vi "value to ring (SequenceNumberOffset).vi"(11 "value":string) -> (3 "SequenceNumberOffset":T1=65535 items=["FDX_TX_FRAME_SEQ_OFFS_AUTO"=65535])   [LabVIEW 2020, in "AIM ARINC 664 Import.lvlib"]
uses:
  AIM ARINC 664 Import.lvlib
  _typedefs/frame_tx_generic_seqNumberOffset.ctl
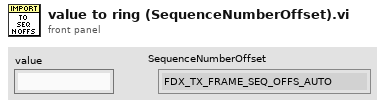
[diagram p1: front panel]
types:
  T1 = typedef "AIM ARINC 664 Import.lvlib/frame_tx_generic_seqNumberOffset.ctl" = i32
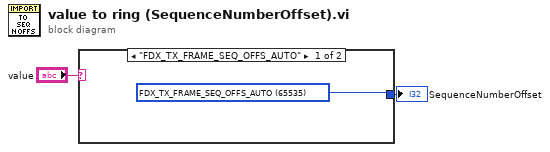
[diagram p0: block diagram]
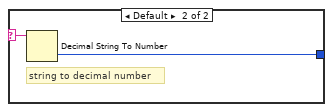
[diagram p2: hidden frame]
diagram:
  n1 = case shown="\"FDX_TX_FRAME_SEQ_OFFS_AUTO\"" "value" {
    selector: "value" -> [_ w5]
    tunnel: [w3 w4] -> w1
    frame "FDX_TX_FRAME_SEQ_OFFS_AUTO" {
      w3 = T1 65535 items=["FDX_TX_FRAME_SEQ_OFFS_AUTO"=65535] ("SequenceNumberOffset")
    }
    frame Default {
      # "string to decimal number"
      n2 = Decimal String To Number(string=w5) -> (number=w4:i32)  [unwired: 2 in, 1 out]
    }
  }
  "SequenceNumberOffset" <- w1
